vi "client state machine.vi"(11 "connection client in":refnum<class "connection client.lvclass">) -> ()   [LabVIEW 2015, in "connection client.lvclass"]
uses:
  connection client.lvclass
  client state.ctl
  connection/connection maintainer.lvclass
  communicator/communicator.lvclass/communicator.ctl
  connection client.lvclass/connection client.ctl
  message/communicator message.lvclass/communicator message.ctl
  communicator/enqueue variety.ctl
  Queue connection/Queue connection.lvclass
  communicator/communicator.lvclass
  message/communicator message.lvclass
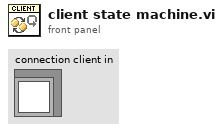
[diagram p1: front panel]
types:
  T1 = typedef "connection maintainer.lvclass/client state.ctl" = enum16{"open", "close", "check queue"}
  T2 = typedef "communicator.lvclass/enqueue variety.ctl" = enum16{"normal", "lossy", "priority"}
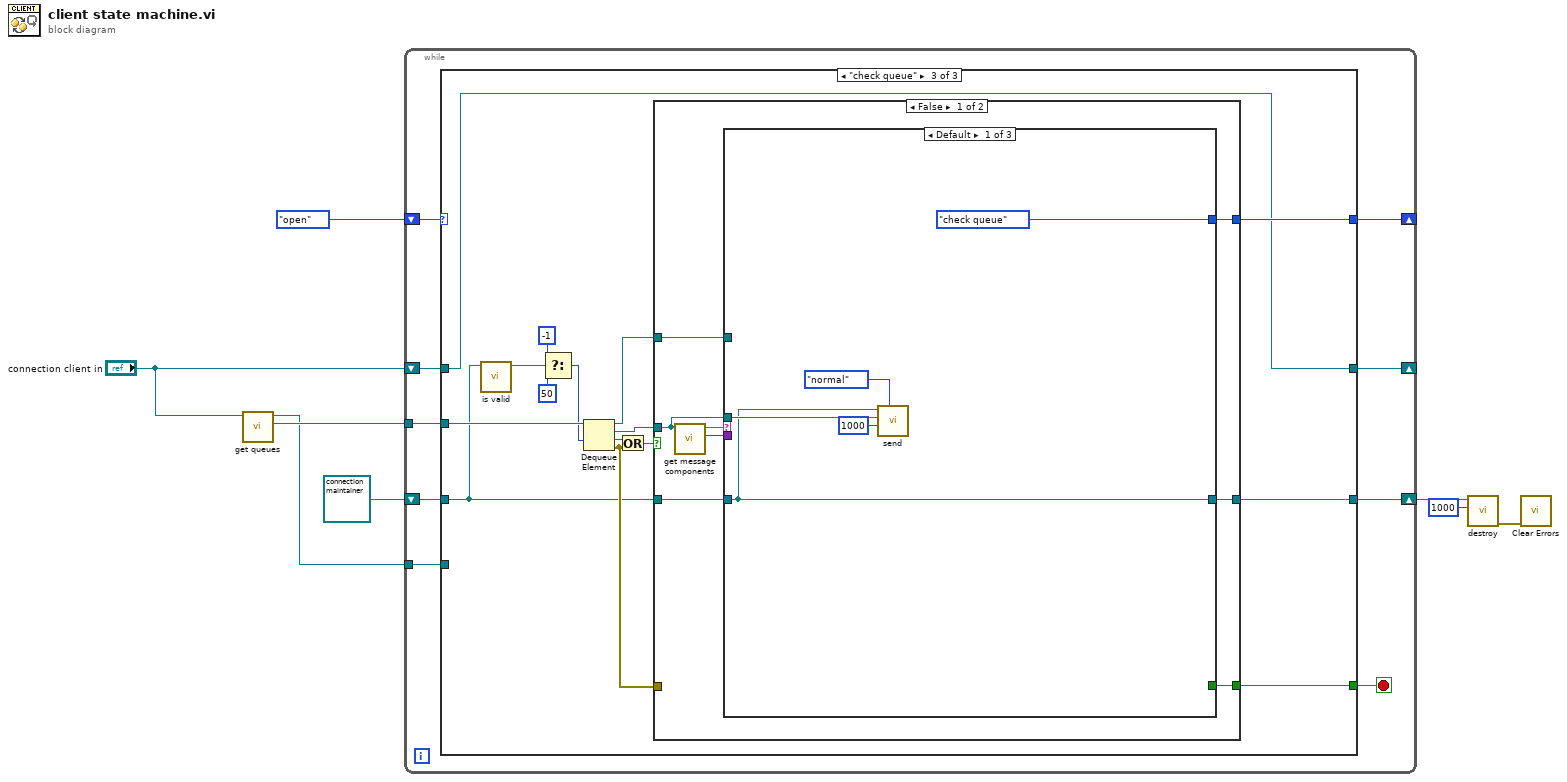
[diagram p0: block diagram]
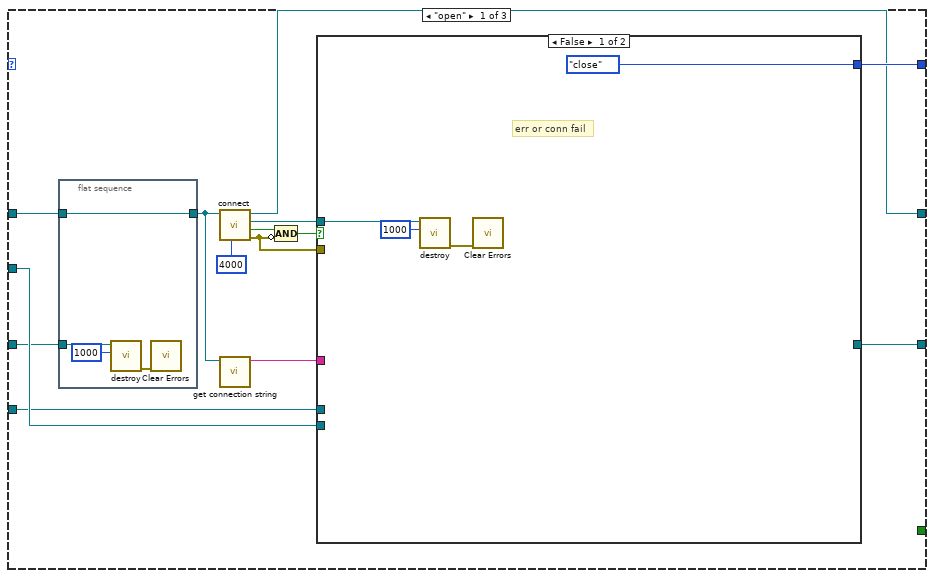
[diagram p2: hidden frame]
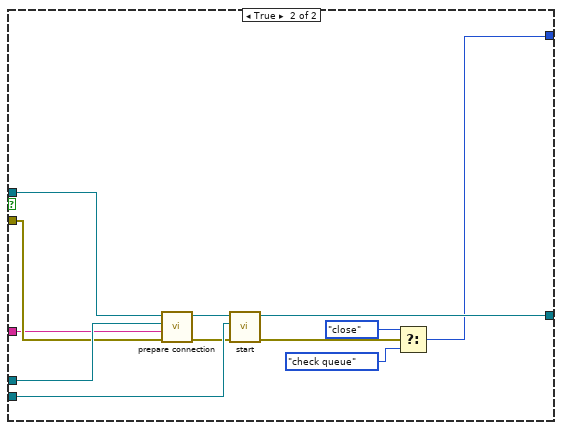
[diagram p3: hidden frame]
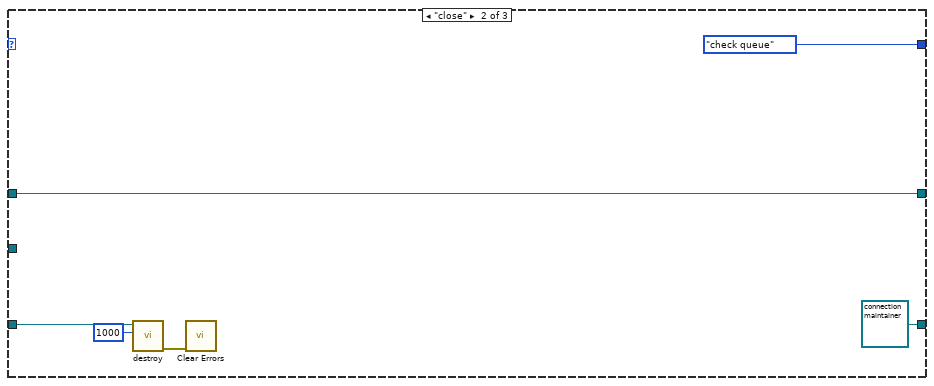
[diagram p4: hidden frame]
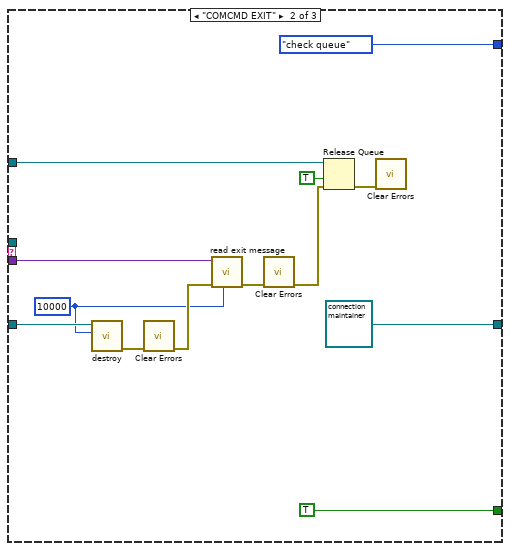
[diagram p5: hidden frame]
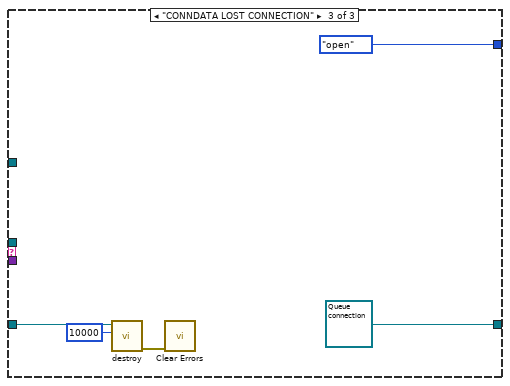
[diagram p6: hidden frame]
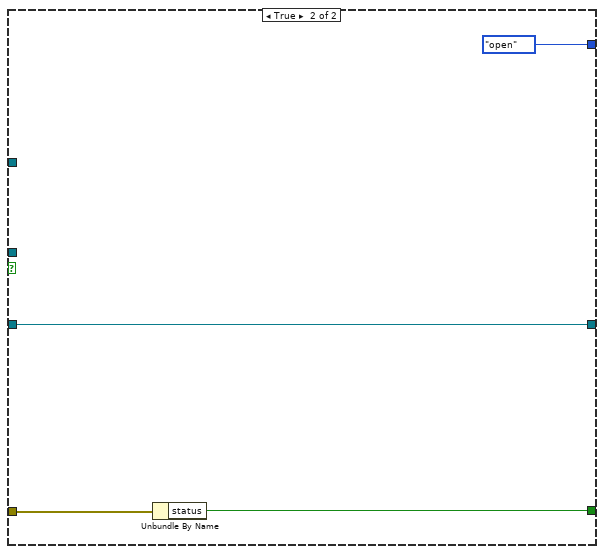
[diagram p7: hidden frame]
diagram:
  n1 = call "get queues.vi"("communicator in"="connection client in") -> ("to worker"=w4:refnum<queue>, "to parent"=w3:refnum<queue>)  [unwired: 9 in]
  n2 = while {
    shift-right: [w16] -> _
    shift-left: client_state."open" -> [w17]
    tunnel: w3 -> [w15]
    tunnel: w4 -> [w14]
    shift-right: [w11] -> w6
    shift-left: refnum<class "connection maintainer.lvclass"> refnum ("connection") -> [w12]
    shift-right: [w9] -> _
    shift-left: "connection client in" -> [w10]
    stop <- w13 stop-if-true
    n3 = case shown="\"check queue\"" w17 {
      tunnel: [w31 client_state."check queue" w67] -> w16
      tunnel: w15 -> [w28 _ _]
      tunnel: w14 -> [w29 _ w72]
      tunnel: [_ _ w68] -> w13
      tunnel: w12 -> [w27 w54 w62]
      tunnel: [w30 refnum<class "connection maintainer.lvclass"> refnum ("connection") w64] -> w11
      tunnel: w10 -> [w25 w53 w63]
      tunnel: [w21 w53 w63] -> w9
      frame "open" {
        n4 = flat-sequence {
          tunnel: w27 -> [w35]
          tunnel: [w32] -> w19
          tunnel: w25 -> [w32]
          frame #0 {
            n5 = call-dynamic "destroy.vi"("timeout in ms (-1)"=1000, "communicator in"=w35) -> ("error out"=w34:errorcluster)  [unwired: 9 in]
            n6 = call <vilib>:"Clear Errors.vi"("error in (no error)"=w34) -> ()  [unwired: 5 in, 2 out]
          }
        }
        n7 = call-dynamic "connect.vi"("timeout ms (10000)"=4000, "connection client in"=w19) -> ("error out"=w24:errorcluster, "valid?"=w23:bool, "new connection"=w22:refnum<class "connection maintainer.lvclass">, "connection client out"=w21:refnum<class "connection client.lvclass">)  [unwired: 6 in]
        n8 = call "get connection string.vi"("connection client in"=w19) -> ("connection string"=w18:string)  [unwired: 10 in]
        n9 = Compound Arithmetic op=AND(w23, invert w24) -> (w26:bool)
        n10 = case shown="False" w26 {
          tunnel: [client_state."close" w47] -> w31
          tunnel: [_ w51] -> w30
          tunnel: w29 -> [_ w46]
          tunnel: w28 -> [_ w44]
          tunnel: w24 -> [_ w43]
          tunnel: w22 -> [w36 w45]
          tunnel: w18 -> [_ w40]
          frame False {
            # "err or conn fail"
            n11 = call-dynamic "destroy.vi"("timeout in ms (-1)"=1000, "communicator in"=w36) -> ("error out"=w37:errorcluster)  [unwired: 9 in]
            n12 = call <vilib>:"Clear Errors.vi"("error in (no error)"=w37) -> ()  [unwired: 5 in, 2 out]
          }
          frame True {
            n13 = call-dynamic "prepare connection.vi"("error in"=w43, "connection string"=w40, "to queue manager"=w44, "connection in"=w45) -> ("error out"=w42:errorcluster, "connection out"=w41:refnum<class "connection maintainer.lvclass">)  [unwired: 6 in]
            n14 = call-dynamic "start.vi"("error in"=w42, "queue to parent"=w46, "communicator in"=w41) -> ("error out"=w50:errorcluster, "communicator out"=w51:refnum<class "connection maintainer.lvclass">)  [unwired: 7 in]
            n15 = Select(t=client_state."close", s=w50, f=client_state."check queue") -> (s? t:f=w47:T1)
          }
        }
      }
      frame "close" {
        n16 = call-dynamic "destroy.vi"("timeout in ms (-1)"=1000, "communicator in"=w54) -> ("error out"=w55:errorcluster)  [unwired: 9 in]
        n17 = call <vilib>:"Clear Errors.vi"("error in (no error)"=w55) -> ()  [unwired: 5 in, 2 out]
      }
      frame "check queue" {
        n18 = call-dynamic "is valid.vi"("connection in"=w62) -> ("valid"=w61:bool)  [unwired: 10 in]
        n19 = Select(t=-1 ("timeout in ms (-1)"), s=w61, f=50 ("timeout in ms (-1)")) -> (s? t:f=w65:i32)
        n20 = Dequeue Element(queue=w72, timeout in ms (-1)=w65) -> (queue out=w58:refnum<queue>, element=w69:refnum<class "communicator message.lvclass">, timed out?=w71:bool, error out=w66:errorcluster)  [unwired: 1 in]
        n21 = Or(x=w71, y=w66) -> (x .or. y?=w70:bool)
        n22 = case shown="False" w70 {
          tunnel: w69 -> [w73 _]
          tunnel: [w80 w105] -> w68
          tunnel: [w77 client_state."open"] -> w67
          tunnel: w66 -> [_ w106]
          tunnel: w62 -> [w78 w104]
          tunnel: [w79 w104] -> w64
          tunnel: w58 -> [w76 _]
          frame False {
            n23 = call "get message components.vi"("message"=w73) -> ("data"=w74:variant, "ID"=w75:string)  [unwired: 9 in]
            n24 = case shown="Default" w75 {
              tunnel: w74 -> [_ w98 _]
              tunnel: [_ TRUE ("element") _] -> w80
              tunnel: [w81 refnum<class "connection maintainer.lvclass"> refnum ("connection") refnum<class "Queue connection.lvclass"> refnum ("TCP connection.lvclass")] -> w79
              tunnel: w78 -> [w81 w94 w101]
              tunnel: [client_state."check queue" client_state."check queue" client_state."open"] -> w77
              tunnel: w76 -> [_ w92 _]
              tunnel: w73 -> [w84 _ _]
              frame Default {
                n25 = call "send.vi"("enqueue setting"=enqueue_variety."normal", "timeout in ms (-1)"=1000, "element"=w84, "communicator in"=w81) -> ()  [unwired: 7 in, 1 out]
              }
              frame "COMCMD EXIT" {
                w87 = 10000 ("timeout in ms (-1)")
                n26 = call-dynamic "destroy.vi"("timeout in ms (-1)"=w87, "communicator in"=w94) -> ("error out"=w95:errorcluster)  [unwired: 9 in]
                n27 = call <vilib>:"Clear Errors.vi"("error in (no error)"=w95) -> ("error out"=w88:errorcluster)  [unwired: 5 in, 1 out]
                n28 = call "read exit message.vi"("timeout in ms (1000)"=w87, "error in"=w88, "data"=w98) -> ("error out"=w90:errorcluster)  [unwired: 8 in]
                n29 = call <vilib>:"Clear Errors.vi"("error in (no error)"=w90) -> ("error out"=w86:errorcluster)  [unwired: 5 in, 1 out]
                n30 = Release Queue(queue=w92, force destroy? (F)=TRUE, error in (no error)=w86) -> (error out=w91:errorcluster)  [unwired: 2 out]
                n31 = call <vilib>:"Clear Errors.vi"("error in (no error)"=w91) -> ()  [unwired: 5 in, 2 out]
              }
              frame "CONNDATA LOST CONNECTION" {
                n32 = call-dynamic "destroy.vi"("timeout in ms (-1)"=10000, "communicator in"=w101) -> ("error out"=w102:errorcluster)  [unwired: 9 in]
                n33 = call <vilib>:"Clear Errors.vi"("error in (no error)"=w102) -> ()  [unwired: 5 in, 2 out]
              }
            }
          }
          frame True {
            n34 = Unbundle By Name(w106) -> ("status"=w105:bool)
          }
        }
      }
    }
  }
  n35 = call-dynamic "destroy.vi"("timeout in ms (-1)"=1000, "communicator in"=w6) -> ("error out"=w7:errorcluster)  [unwired: 9 in]
  n36 = call <vilib>:"Clear Errors.vi"("error in (no error)"=w7) -> ()  [unwired: 5 in, 2 out]
